vi "Report-AllComics.vi"() -> ()   [LabVIEW 2022 SP3]
uses:
  TypeDefs/Comic.ctl
  TypeDefs/Character.ctl
  TypeDefs/Creator.ctl
  TypeDefs/Variant.ctl
panel:
  out "Current Comic":string
  out "appended array":string[][](array[string])
  in  "ComicsRootPath":path=path "C:/data/comics/comics"
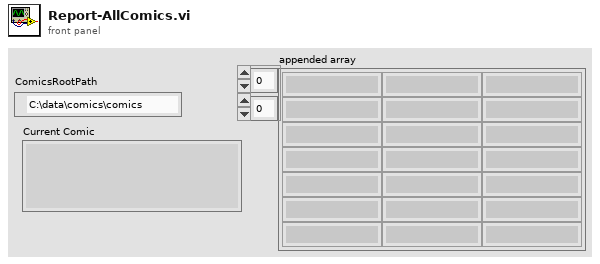
[diagram p1: front panel]
types:
  T1 = typedef "Comic.ctl" = cluster{"URL":string, "Series URL":string, "Series":string, "Volume":i32, "Issue":string, "Title":string, "Description":string, "Page Count":i32, "Cover Price":dbl, "UPC":string, "Characters":T2[], "Creators":T3[], "Main Cover URL":string, "Variant Covers":T4[], "DatePublished":timestamp}
  T2 = typedef "Character.ctl" = cluster{"Name":string, "Real-Name":string, "Universe":string, "URL":string}
  T3 = typedef "Creator.ctl" = cluster{"Name":string, "URL":string, "Creator Types":string[]}
  T4 = typedef "Variant.ctl" = cluster{"URL":string, "Description":string, "Cover URL":string}
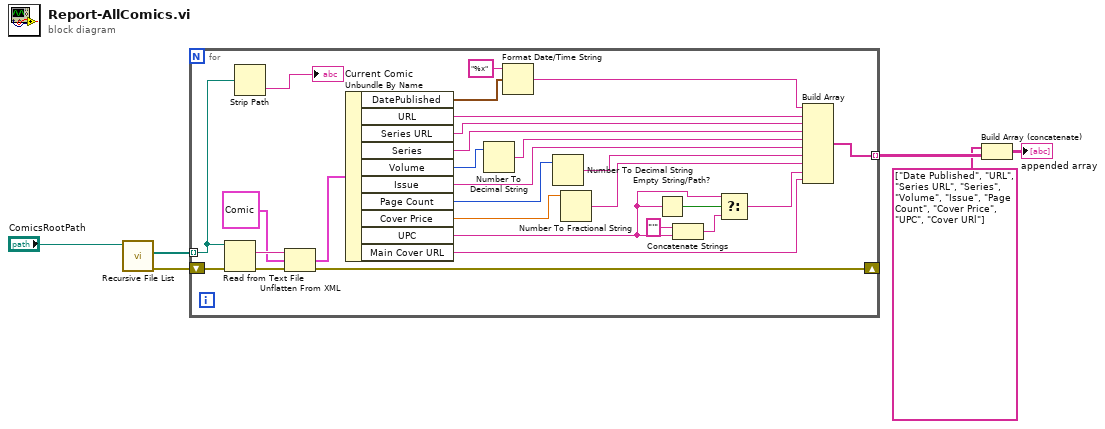
[diagram p0: block diagram]
diagram:
  n1 = call <vilib>:"Recursive File List.vi"("Folder Path"="ComicsRootPath") -> ("error out"=w4:errorcluster, "All Files in Dir"=w5:path[])  [unwired: 6 in, 3 out]
  n2 = for {
    tunnel: w5 -> [w13] mode=indexing
    shift-right: [w29] -> _
    shift-left: w4 -> [w34]
    tunnel: [w17] -> w3 mode=indexing
    n3 = Read from Text File(file (use dialog)=w13, error in=w34) -> (text=w32:string, error out=w33:errorcluster)  [unwired: 2 in, 2 out]
    n4 = Strip Path(path=w13) -> (name=→"Current Comic":string)  [unwired: 1 out]
    n5 = Unflatten From XML(xml string=w32, type=T1 {"URL"="", "Series URL"="", "Series"="", "Volume"=0, "Issue"="", "Title"="", "Description"="", "Page Count"=0, "Cover Price"=0.0, "UPC"="", "Characters"=[], "Creators"=[], "Main Cover URL"="", "Variant Covers"=[], "DatePublished"=timestamp(0 s since 1904-01-01)} ("Comic"), error in (no error)=w33) -> (value=w30:T1, error out=w29:errorcluster)
    n6 = Unbundle By Name(w30) -> ("DatePublished"=w16:timestamp, "URL"=w25:string, "Series URL"=w24:string, "Series"=w23:string, "Volume"=w28:i32, "Issue"=w21:string, "Page Count"=w27:i32, "Cover Price"=w26:dbl, "UPC"=w8:string, "Main Cover URL"=w18:string)
    n7 = Number To Decimal String(number=w28) -> (decimal integer string=w22:string)  [unwired: 1 in]
    n8 = Format Date/Time String(time format string (%c)="%x", seconds (now)=w16) -> (date/time string=w15:string)  [unwired: 1 in]
    n9 = Number To Decimal String(number=w27) -> (decimal integer string=w20:string)  [unwired: 1 in]
    n10 = Number To Fractional String(number=w26) -> (F-format string=w19:string)  [unwired: 3 in]
    n11 = Empty String/Path?(string/path=w8) -> (empty?=w9:bool)
    n12 = Concatenate Strings("'" ("string"), w8) -> (w10:string)
    n13 = Select(t=w8, s=w9, f=w10) -> (s? t:f=w7:string)
    n14 = Build Array(w15, w25, w24, w23, w22, w21, w20, w19, w7, w18) -> (w17:string[])
  }
  n15 = Build Array (concatenate)(string[] ["Date Published", "URL", "Series URL", "Series", "Volume", "Issue", "Page Count", "Cover Price", "UPC", "Cover URl"], w3) -> (→"appended array":string[][])
